vi "7SPOTMEASnov.vi"() -> ()   [LabVIEW 2020]
panel:
  in  "Channel":i32
  in  "VISA resource name":refnum<visa-resource-name>
  out "Measurement Result":dbl
  in  "Measurement Mode (0:Voltage)":enum16{"Voltage", "Current", "Resistance"}(ring)
  # "CURRENT IN mA\nVOLTAGE IN V\nRESISTANCE IN Ohms"
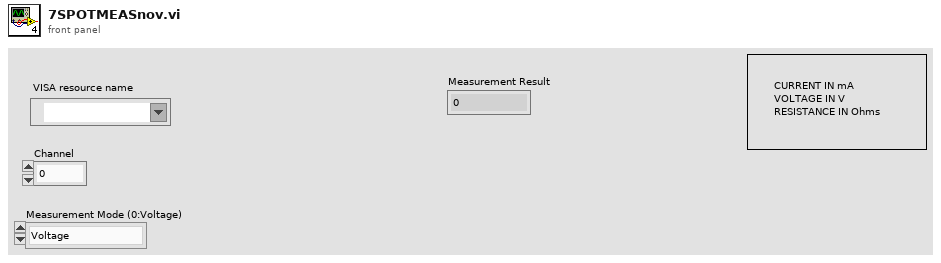
[diagram p1: front panel]
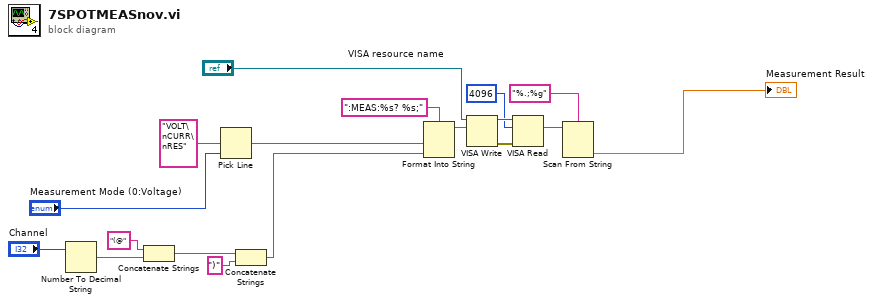
[diagram p0: block diagram]
diagram:
  n1 = Number To Decimal String(number="Channel") -> (decimal integer string=w5:string)  [unwired: 1 in]
  n2 = Concatenate Strings("(@", w5) -> (w4:string)
  n3 = Pick Line(multi-line string="VOLT\nCURR\nRES", line index="Measurement Mode (0:Voltage)") -> (output string=w15:string)  [unwired: 1 in]
  n4 = Concatenate Strings(w4, ")") -> (w2:string)
  n5 = Format Into String(format string=":MEAS:%s? %s;", w15, w2) -> (resulting string=w12:string)  [unwired: 2 in, 1 out]
  n6 = VISA Write(VISA resource name="VISA resource name", write buffer=w12) -> (VISA resource name out=w9:refnum<visa-resource-name>, error out=w10:errorcluster)  [unwired: 1 in, 1 out]
  n7 = VISA Read(VISA resource name=w9, byte count=u32 4096, error in (no error)=w10) -> (read buffer=w18:string)  [unwired: 3 out]
  n8 = Scan From String(format string="%.;%g", input string=w18) -> (output 1=→"Measurement Result":dbl)  [unwired: 3 in, 3 out]
